vi "trplot.vi"(8 "Error In":errorcluster, 9 "theta":dbl, 10 "y":dbl, 11 "x":dbl) -> (0 "Error Out":errorcluster, 3 "t":dbl[][](array[numeric]))   [LabVIEW 2013]
doc: "This function builds and outputs a 3x3 homogeneous transformation as a 2-D array(t). Inputs are horizontal translation (X), vertical translation (Y), and rotation (theta) in radians. The default value of theta is 0 rad."
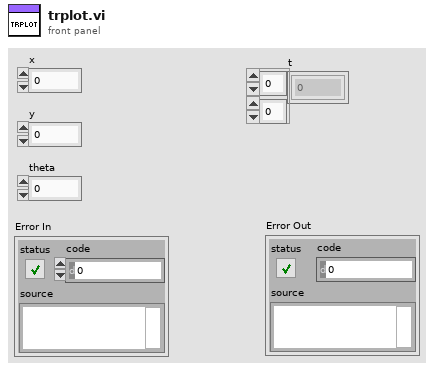
[diagram p1: front panel]
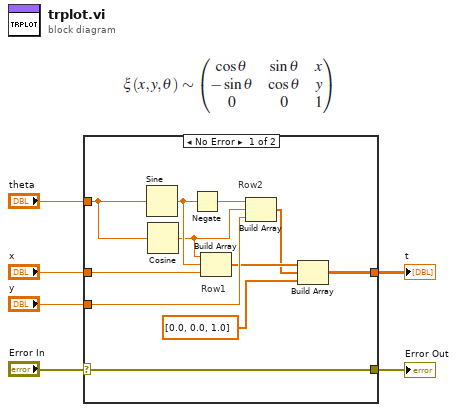
[diagram p0: block diagram]
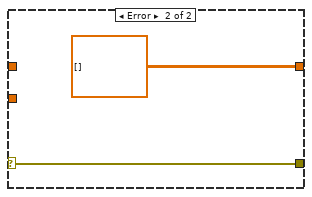
[diagram p2: hidden frame]
diagram:
  n1 = case shown="No Error" "Error In" {
    selector: "Error In" -> [w17 w18]
    tunnel: [w17 w18] -> w5
    tunnel: "x" -> [w15 _]
    tunnel: "y" -> [w11 _]
    tunnel: "theta" -> [w16 _]
    tunnel: [w7 dbl[][] [] ("t")] -> w1
    frame No Error {
      # "Row1"
      # "Row2"
      n2 = Sine(x=w16) -> (sin(x)=w13:dbl)
      n3 = Cosine(x=w16) -> (cos(x)=w12:dbl)
      n4 = Negate(x=w13) -> (-x=w14:dbl)
      n5 = Build Array(w12, w13, w15) -> (w10:dbl[])
      n6 = Build Array(w14, w12, w11) -> (w9:dbl[])
      n7 = Build Array(w10, w9, dbl[] [0.0, 0.0, 1.0] ("appended array")) -> (w7:dbl[][])
    }
    frame Error {
    }
  }
  "Error Out" <- w5
  "t" <- w1
